vi "fg_height_width_multiplier.vi"(10 "multiplier":u32=2, 11 "width_height in":u32) -> (3 "width_height out":u32)   [LabVIEW 2015, in "lv-graph.lvlib"]
uses:
  lv-graph.lvlib
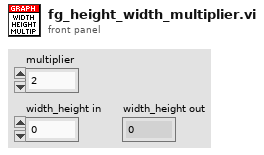
[diagram p1: front panel]
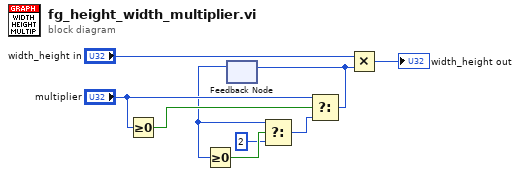
[diagram p0: block diagram]
diagram:
  n1 = Greater Or Equal To 0?(x="multiplier") -> (x >= 0?=w5:bool)
  n2 = feedback #1() -> (w3:u32)  [unwired: 1 in]
  n3 = Greater Or Equal To 0?(x=w3) -> (x >= 0?=w4:bool)
  n4 = Select(t=w3, s=w4, f=u32 2) -> (s? t:f=w1:u32)
  n5 = Select(t="multiplier", s=w5, f=w1) -> (s? t:f=w6:u32)
  n6 = feedback-in #1(w6) -> ()
  n7 = Multiply(x="width_height in", y=w6) -> (x*y=→"width_height out":u32)
